vi "Format Tables.vi"(0 "Header":string[](array[string]), 5 "Data Table":dbl[][](array[numeric])) -> (4 "spreadsheet string":string)   [LabVIEW 2010]
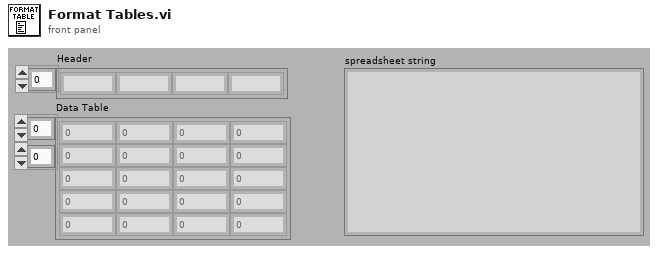
[diagram p1: front panel]
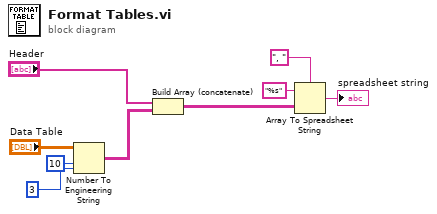
[diagram p0: block diagram]
diagram:
  n1 = Number To Engineering String(2:i16 3 ("precision (6)"), 3:i16 10 ("width (-)"), 4:"Data Table") -> (0:w7:string[][])  [unwired: 1 in]
  n2 = Build Array (concatenate)("Header", w7) -> (w5:string[][])
  n3 = Array To Spreadsheet String(delimiter (Tab)=", ", array=w5, 3:"%s" ("format string")) -> (spreadsheet string=→"spreadsheet string":string)
